vi "Connect Tunnels.vi"(8 "targetID":string, 10 "orig tsRef":refnum<vi>, 11 "inst tsRef":refnum<vi>) -> (2 "orig tsRef out":refnum<vi>)   [LabVIEW 2020, in "NI_TargetHelper.lvlib"]
uses:
  <vilib>/TargetSupport/NI_TargetHelper/NI_TargetHelper.lvlib
  <vilib>/Utility/miscctls.llb/LVPositionTypeDef.ctl
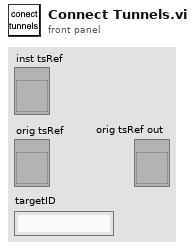
[diagram p1: front panel]
types:
  T1 = typedef "LVPositionTypeDef.ctl" = cluster{"Left":i32, "Top":i32}
  T2 = typedef "NI_TargetHelper.lvlib/Instance VIref.ctl" = refnum<vi>
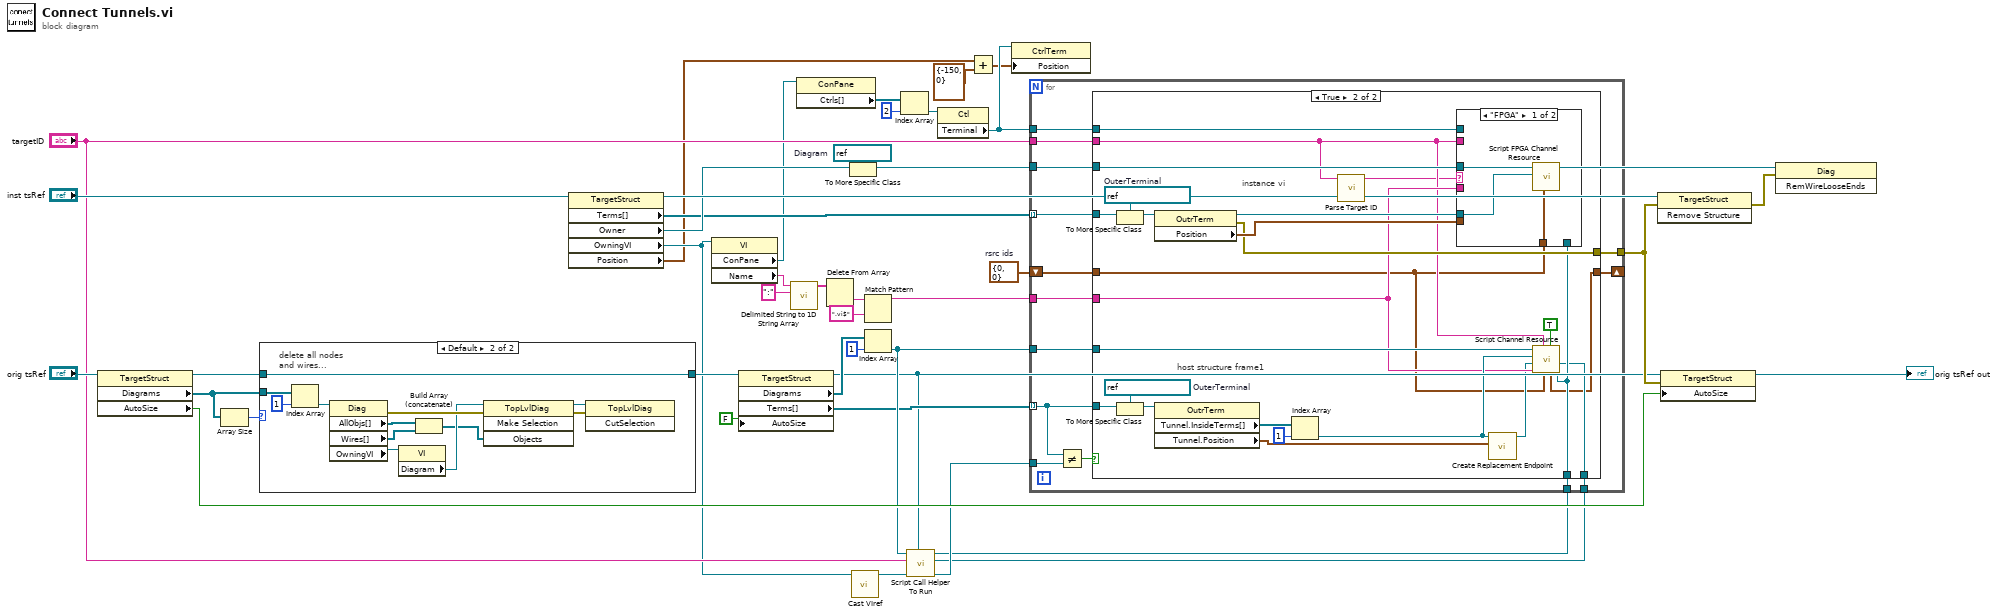
[diagram p0: block diagram]
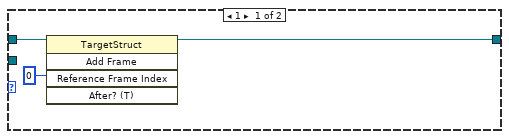
[diagram p2: hidden frame]
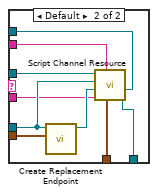
[diagram p4: hidden frame]
diagram:
  w31 = cluster{"tag":u32, "stream":u32} {"tag"=0, "stream"=0}  # rsrc ids
  w40 = refnum<vi> refnum  # Diagram
  n1 = property class="TargetStruct"(reference="orig tsRef") -> (reference out=w36:refnum<vi>, "Diagrams"=w23:refnum<vi>[], "AutoSize"=w28:bool)  [unwired: 1 in, 1 out]
  n2 = Array Size(array=w23) -> (size(s)=w35:i32)
  n3 = case shown="Default" w35 {
    tunnel: [w44 w57] -> w37
    tunnel: w36 -> [w43 w57]
    tunnel: w23 -> [_ w56]
    frame 1 {
      n4 = invoke class="TargetStruct" method="Add Frame"(reference=w43, "Reference Frame Index"=u32 0) -> (reference out=w44:refnum<vi>)  [unwired: 3 in, 4 out]
    }
    frame Default {
      # "delete all nodes\nand wires..."
      n5 = Index Array(array=w56, index=1) -> (element=w50:refnum<vi>)
      n6 = property class="Diag"(reference=w50) -> (error out=w52:errorcluster, "AllObjs[]"=w54:refnum<vi>[], "Wires[]"=w46:refnum<vi>[], "OwningVI"=w49:refnum<vi>)  [unwired: 1 in, 1 out]
      n7 = property class="VI"(reference=w49) -> ("Diagram"=w48:refnum<vi>)  [unwired: 1 in, 2 out]
      n8 = Build Array (concatenate)(w54, w46) -> (w47:refnum<vi>[])
      n9 = invoke class="TopLvlDiag" method="Make Selection"(reference=w48, error in=w52, "Objects"=w47) -> (reference out=w53:refnum<vi>, error out=w51:errorcluster)  [unwired: 1 in, 2 out]
      n10 = invoke class="TopLvlDiag" method="CutSelection"(reference=w53, error in=w51) -> ()  [unwired: 1 in, 3 out]
    }
  }
  n11 = property class="TargetStruct"(reference="inst tsRef") -> (reference out=w42:refnum<vi>, "Terms[]"=w32:refnum<vi>[], "Owner"=w33:refnum<vi>, "OwningVI"=w13:refnum<vi>, "Position"=w4:T1)  [unwired: 1 in, 1 out]
  n12 = property class="VI"(reference=w13) -> ("ConPane"=w9:refnum<vi>, "Name"=w20:string)  [unwired: 1 in, 2 out]
  n13 = property class="TargetStruct"(reference=w37, "AutoSize"=FALSE ("AutoSize To Fit Contents?")) -> (reference out=w11:refnum<vi>, "Diagrams"=w30:refnum<vi>[], "Terms[]"=w15:refnum<vi>[])  [unwired: 1 in, 1 out]
  n14 = call <vilib>:"Delimited String to 1D String Array.vi"("delimiter"=":", "delimited string"=w20) -> ("string array"=w19:string[])  [unwired: 9 in]
  n15 = property class="ConPane"(reference=w9) -> ("Ctrls[]"=w8:refnum<vi>[])  [unwired: 1 in, 2 out]
  n16 = Delete From Array(array=w19) -> (deleted portion=w18:string)  [unwired: 2 in, 1 out]
  n17 = To More Specific Class(target class=w40, reference=w33) -> (specific class reference=w38:refnum<vi>)  [unwired: 1 in, 1 out]
  n18 = call <vilib>:"Cast VIref.vi"("VI Refnum"=w13) -> ("instVIref"=w12:T2)  [unwired: 10 in]
  n19 = Match Pattern(string=w18, regular expression=".vi$") -> (before substring=w21:string)  [unwired: 1 in, 3 out]
  n20 = Index Array(array=w30, index=1) -> (element=w25:refnum<vi>)
  n21 = Index Array(array=w8, index=2) -> (element=w6:refnum<vi>)
  n22 = call <vilib>:"Script Call Helper To Run.vi"("orig tsRef"=w11, "instVIref"=w12, "targetID"="targetID", "diagram"=w25) -> ("addr term"=w16:refnum<vi>, "clone term"=w10:refnum<vi>, "target object term"=w14:refnum<vi>)  [unwired: 5 in]
  n23 = property class="Ctl"(reference=w6) -> ("Terminal"=w5:refnum<vi>)  [unwired: 1 in, 2 out]
  n24 = Add(x=w4, y=T1 {"Left"=-150, "Top"=0}) -> (x+y=w3:T1)
  n25 = property class="CtrlTerm"(reference=w5, "Position"=w3) -> ()  [unwired: 1 in, 2 out]
  n26 = for {
    tunnel: w32 -> [w71] mode=indexing
    tunnel: [w70] -> w27
    shift-right: [w66] -> _
    shift-left: w31 -> [w65]
    tunnel: w38 -> [w69]
    tunnel: "targetID" -> [w67]
    tunnel: w25 -> [w68]
    tunnel: w15 -> [w58] mode=indexing
    tunnel: w21 -> [w64]
    tunnel: w16 -> [w62]
    tunnel: w14 -> [w61]
    tunnel: w10 -> [w60]
    tunnel: w5 -> [w59]
    n27 = Not Equal?(x=w58, y=w62) -> (x != y?=w63:bool)
    n28 = case shown="True" w63 {
      tunnel: w71 -> [_ w97]
      tunnel: [_ w93] -> w70
      tunnel: w58 -> [_ w88]
      tunnel: w69 -> [_ w87]
      tunnel: w68 -> [_ w85]
      tunnel: w67 -> [_ w76]
      tunnel: [w72 w74] -> w66
      tunnel: w65 -> [w72 w73]
      tunnel: w64 -> [_ w82]
      tunnel: w61 -> [_ w79]
      tunnel: w60 -> [_ w78]
      tunnel: w59 -> [_ w77]
      frame False {
        # "skip addr terminal since it isn't a channel"
      }
      frame True {
        w91 = refnum<vi> refnum  # OuterTerminal
        w95 = refnum<vi> refnum  # OuterTerminal
        # "instance vi"
        # "host structure frame1"
        n29 = To More Specific Class(target class=w95, reference=w97) -> (specific class reference=w96:refnum<vi>)  [unwired: 1 in, 1 out]
        n30 = To More Specific Class(target class=w91, reference=w88) -> (specific class reference=w90:refnum<vi>)  [unwired: 1 in, 1 out]
        n31 = property class="OutrTerm"(reference=w96) -> (reference out=w86:refnum<vi>, error out=w93:errorcluster, "Position"=w94:T1)  [unwired: 1 in]
        n32 = property class="OutrTerm"(reference=w90) -> ("Tunnel.InsideTerms[]"=w89:refnum<vi>[], "Tunnel.Position"=w84:T1)  [unwired: 1 in, 2 out]
        n33 = Index Array(array=w89, index=1) -> (element=w83:refnum<vi>)
        n34 = call <vilib>:"Parse Target ID.vi"("targetID"=w76) -> ("target name"=w75:string)  [unwired: 9 in, 1 out]
        n35 = case shown="\"FPGA\"" w75 {
          tunnel: w94 -> [_ w109]
          tunnel: w87 -> [w98 w108]
          tunnel: w86 -> [w100 w107]
          tunnel: w76 -> [_ w105]
          tunnel: w73 -> [w99 w104]
          tunnel: w82 -> [_ w103]
          tunnel: w79 -> [_ w102]
          tunnel: w77 -> [_ w101]
          frame "FPGA" {
            n36 = call <vilib>:"Script FPGA Channel Resource.vi"("rsrc ids in"=w99, "tunnel term"=w100, "diagram"=w98) -> ()  [unwired: 9 in]
          }
          frame Default {
            n37 = call <vilib>:"Create Replacement Endpoint.vi"("position"=w109, "tunnel term"=w107) -> ("endpt"=w106:refnum<vi>)  [unwired: 7 in]
            n38 = call <vilib>:"Script Channel Resource.vi"("target object term"=w102, "clone term"=w101, "rsrc ids in"=w104, "targetID"=w105, "prefix"=w103, "endpt"=w106, "tunnel term"=w107, "diagram"=w108) -> ()  [unwired: 3 in, 1 out]
          }
        }
        n39 = call <vilib>:"Create Replacement Endpoint.vi"("position"=w84, "tunnel term"=w83) -> ("endpt"=w81:refnum<vi>)  [unwired: 7 in]
        n40 = call <vilib>:"Script Channel Resource.vi"("target object term"=w79, "clone term"=w78, "host frame1"=TRUE, "rsrc ids in"=w73, "targetID"=w76, "prefix"=w82, "endpt"=w81, "tunnel term"=w83, "diagram"=w85) -> ("rsrc ids out"=w74:cluster{"tag":u32, "stream":u32})  [unwired: 2 in]
      }
    }
  }
  n41 = invoke class="TargetStruct" method="Remove Structure"(reference=w42, error in=w27) -> (error out=w39:errorcluster)  [unwired: 1 in, 2 out]
  n42 = property class="TargetStruct"(reference=w11, error in=w27, "AutoSize"=w28) -> (reference out=→"orig tsRef out":refnum<vi>)  [unwired: 1 out]
  n43 = invoke class="Diag" method="RemWireLooseEnds"(reference=w38, error in=w39) -> ()  [unwired: 1 in, 3 out]
